vi "Multiply Polynomials (CDB).vi"(8 "threshold type":T1 items=["Absolute Value", "Relative Value"], 9 "threshold":dbl, 10 "Q(x)":cdb[](array[numeric]) format="%#.6g", 11 "P(x)":cdb[](array[numeric]) format="%#.6g") -> (0 "error":i32, 3 "P(x)*Q(x)":cdb[](array[numeric]) format="%#.6g")   [LabVIEW 2020, in "NI_AALPro.lvlib"]
doc: "Multiplies polynomial <B>P(x)</B> by polynomial <B>Q(x)</B>. The data types you wire to the <B>P(x)</B> and <B>Q(x)</B> inputs determine the polymorphic instance to use."
uses:
  NI_AALPro.lvlib
  Remove Zero Threshold Type.ctl
  Remove Zero Coefficients (CDB).vi
  <resource>/lvanlys.dll
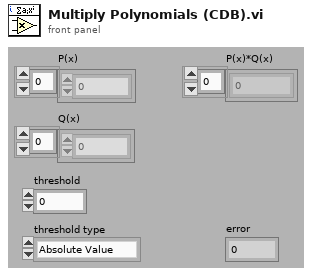
[diagram p1: front panel]
types:
  T1 = typedef "NI_AALPro.lvlib/Remove Zero Threshold Type.ctl" = u16
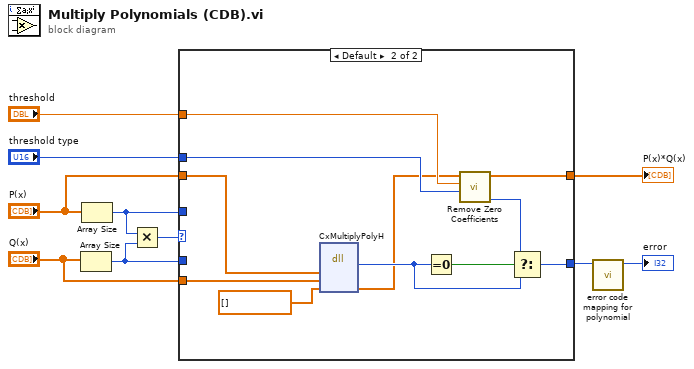
[diagram p0: block diagram]
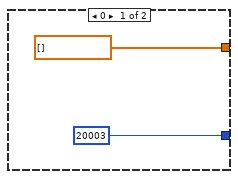
[diagram p2: hidden frame]
diagram:
  n1 = Array Size(array="Q(x)") -> (size(s)=w6:i32)
  n2 = Array Size(array="P(x)") -> (size(s)=w7:i32)
  n3 = Multiply(x=w7, y=w6) -> (x*y=w8:i32)
  n4 = case shown="Default" w8 {
    tunnel: w7 -> [_ _]
    tunnel: w6 -> [_ _]
    tunnel: "P(x)" -> [_ w17]
    tunnel: "Q(x)" -> [_ w16]
    tunnel: [cdb[] [] ("CDB") w21] -> w5
    tunnel: [20003 ("empty array") w20] -> w4
    tunnel: "threshold type" -> [_ w19]
    tunnel: "threshold" -> [_ w18]
    frame 0 {
    }
    frame Default {
      n5 = dll-call lib="C:/Program Files (x86)/National Instruments/LabVIEW 2020/resource/lvanlys.*" fn="CxMultiplyPolyH"("pH"=w17, "qH"=w16, "pqH"=cdb[] [] ("Q(x)")) -> ("error"=w15:i32, "pqH"=w14:cdb[])  [unwired: 5 in, 2 out]
      n6 = Equal To 0?(x=w15) -> (x = 0?=w23:bool)
      n7 = call-poly "Remove Zero Coefficients.vi"("threshold type"=w19, "threshold"=w18, "P(x) In"=w14) -> ("error"=w22:i32, "P(x) Out"=w21:cdb[])  [unwired: 6 in, 1 out]
      n8 = Select(t=w22, s=w23, f=w15) -> (s? t:f=w20:i32)
    }
  }
  "P(x)*Q(x)" <- w5
  n9 = call "error code mapping for polynomial.vi"("error in"=w4) -> ("error out"=→"error":i32)  [unwired: 10 in]
